vi "viewer.vi"() -> ()   [LabVIEW 2013, in "testmod runtime.lvclass"]
uses:
  testmod runtime.lvclass
panel:
  in  "stop":bool
  out "10k":string
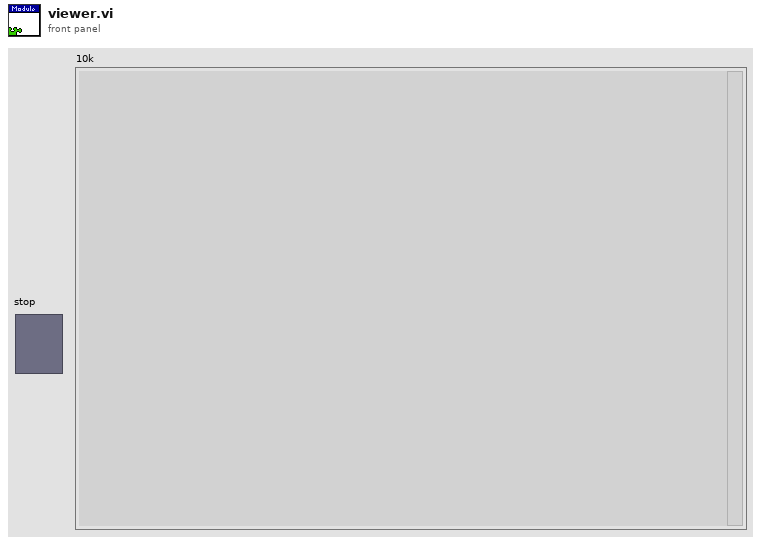
[diagram p1: front panel]
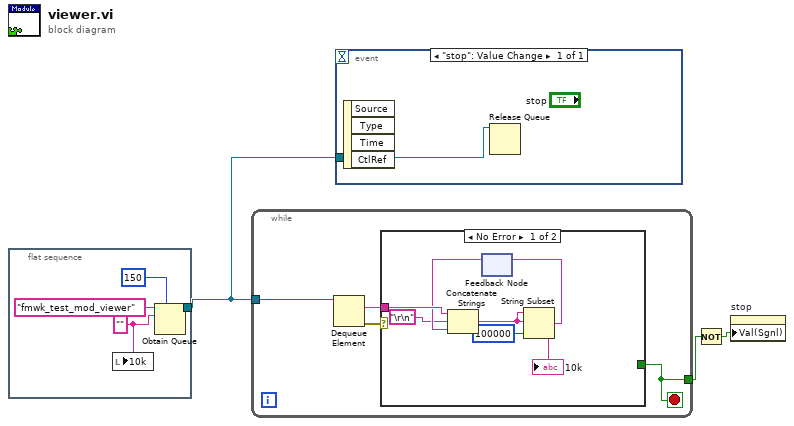
[diagram p0: block diagram]
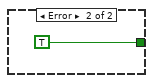
[diagram p2: hidden frame]
diagram:
  n1 = flat-sequence {
    tunnel: [w7] -> w3
    frame #0 {
      w5 = ""
      n2 = local write "10k"(w5) -> ()
      n3 = Obtain Queue(max queue size (-1, unlimited)=150, name (unnamed)="fmwk_test_mod_viewer", element data type=w5) -> (queue out=w7:refnum<queue>)  [unwired: 2 in, 2 out]
    }
  }
  n4 = while {
    tunnel: w3 -> [w11]
    tunnel: [w8] -> w1
    stop <- w8 stop-if-true
    n5 = Dequeue Element(queue=w11) -> (element=w9:string, error out=w10:errorcluster)  [unwired: 2 in, 2 out]
    n6 = case shown="No Error" w10 {
      tunnel: w9 -> [w14 _]
      tunnel: [_ TRUE] -> w8
      frame No Error {
        n7 = feedback #1() -> (w13:string)  [unwired: 1 in]
        n8 = Concatenate Strings(w14, "\r\n", w13) -> (w17:string)
        "10k" <- w17
        n9 = String Subset(string=w17, length (rest)=100000 ("length (rest)")) -> (substring=w16:string)  [unwired: 1 in]
        n10 = feedback-in #1(w16) -> ()
      }
      frame Error {
      }
    }
  }
  n11 = event shown="[0] \"stop\": Value Change" {
    selector: _ -> [_]
    dyn-events: _ -> [_]
    timeout: _ -> [_]
    tunnel: w3 -> [w19]
    event "stop": Value Change {
      n12 = event-data() -> ()  [unwired: 1 in, 4 out]
      n13 = Release Queue(queue=w19) -> ()  [unwired: 2 in, 3 out]
    }
  }
  n14 = Not(x=w1) -> (.not. x?=w2:bool)
  n15 = property on="stop" class="Bool (strict)"("Val(Sgnl)"=w2) -> ()  [unwired: 2 in, 2 out]
